vi "Attenuator_ReadPos.vi"(5 "Axis":u16) -> (1 "Pos out":dbl, 2 "Puls out":i32)   [LabVIEW 2018]
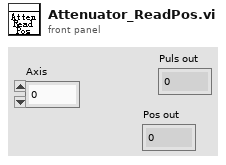
[diagram p1: front panel]
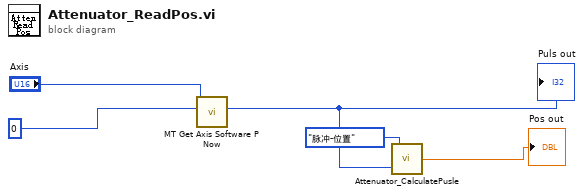
[diagram p0: block diagram]
diagram:
  n1 = call "MT Get Axis Software P Now.vi"("pValue"=0, "AObj"="Axis") -> ("pValue out"=w2:i32)  [unwired: 7 in, 2 out]
  "Puls out" <- w2
  n2 = call "Attenuator_CalculatePusle.vi"("计算状态"=enum32{"位置-脉冲", "脉冲-位置"}."脉冲-位置", "数据"=w2) -> ("dataout"=→"Pos out":dbl)  [unwired: 2 in]
